vi "3D-Conform PosValue.vi"(11 "Pos Set":string[][](table)) -> (3 "输出簇":T1)   [LabVIEW 2011]
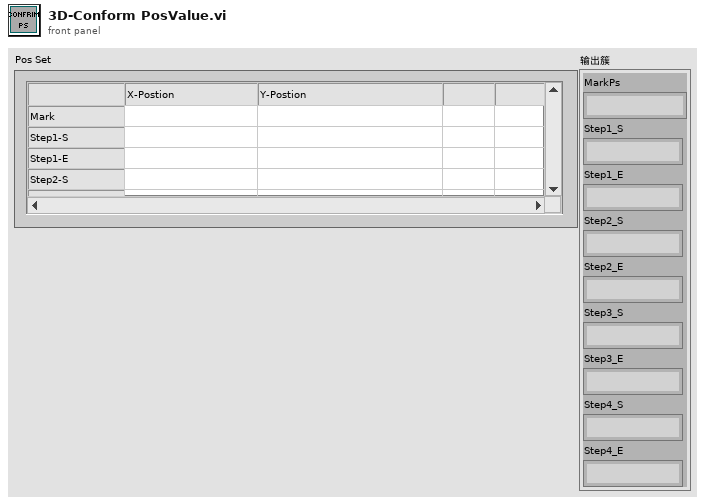
[diagram p1: front panel]
types:
  T1 = cluster{"MarkPs":string, "Step1_S":string, "Step1_E":string, "Step2_S":string, "Step2_E":string, "Step3_S":string, "Step3_E":string, "Step4_S":string, "Step4_E":string}
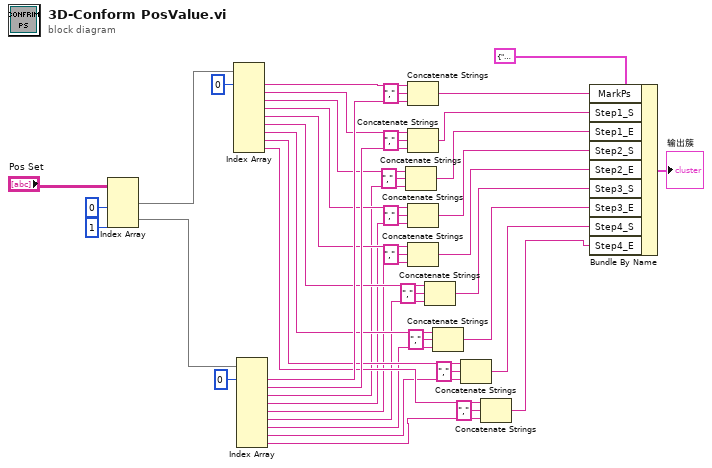
[diagram p0: block diagram]
diagram:
  n1 = Index Array(array="Pos Set", index (col) #1=0 ("禁用的索引 (列)"), index (col) #2=1 ("索引 (列)")) -> (element #1=w39:string[], element #2=w44:string[])  [unwired: 2 in]
  n2 = Index Array(array=w39, index #1=0 ("索引")) -> (element #1=w38:string, element #2=w33:string, element #3=w28:string, element #4=w25:string, element #5=w22:string, element #6=w19:string, element #7=w16:string, element #8=w13:string, element #9=w10:string)  [unwired: 8 in]
  n3 = Index Array(array=w44, index #1=0 ("索引")) -> (element #1=w36:string, element #2=w32:string, element #3=w7:string, element #4=w6:string, element #5=w5:string, element #6=w4:string, element #7=w3:string, element #8=w2:string, element #9=w1:string)  [unwired: 8 in]
  n4 = Concatenate Strings(w28, "," ("字符串"), w7) -> (w27:string)
  n5 = Concatenate Strings(w38, "," ("字符串"), w36) -> (w34:string)
  n6 = Concatenate Strings(w33, "," ("字符串"), w32) -> (w31:string)
  n7 = Concatenate Strings(w25, "," ("字符串"), w6) -> (w23:string)
  n8 = Concatenate Strings(w22, "," ("字符串"), w5) -> (w21:string)
  n9 = Concatenate Strings(w19, "," ("字符串"), w4) -> (w17:string)
  n10 = Concatenate Strings(w16, "," ("字符串"), w3) -> (w14:string)
  n11 = Concatenate Strings(w13, "," ("字符串"), w2) -> (w12:string)
  n12 = Concatenate Strings(w10, "," ("字符串"), w1) -> (w9:string)
  n13 = Bundle By Name(cluster=T1 {"MarkPs"="", "Step1_S"="", "Step1_E"="", "Step2_S"="", "Step2_E"="", "Step3_S"="", "Step3_E"="", "Step4_S"="", "Step4_E"=""} ("parameter Input"), "MarkPs"=w34, "Step1_S"=w31, "Step1_E"=w27, "Step2_S"=w23, "Step2_E"=w21, "Step3_S"=w17, "Step3_E"=w14, "Step4_S"=w12, "Step4_E"=w9) -> (→"输出簇":T1)
